vi "UHR-Fleezers Control (host) - 10.5.vi"() -> ()   [LabVIEW 2011] (continued)
      n139 = xnode "Read/Write Control"("FPGA VI Reference In"=w286, "error in"=w285, "+ phase"=w284, "+ phase (GI)"=w284, "+ phase (MCL)"=w284, "+ phase (APD Acq)"=w284, "+ phase (APD 1 Gate)"=w284, "+ phase (APD 2 Gate)"=w284, "+ phase (Green FB)"=w284, "+ phase (GI) 2"=w284) -> ("FPGA VI Reference Out"=w287:T19, "error out"=w288:errorcluster)
    }
    frame #3 {
      n140 = Wait (ms)(milliseconds to wait=u32 100) -> ()  [unwired: 1 out]
    }
  }
  n141 = local read "Phase adj. (Green FB)"() -> (w117:i16)
  n142 = local read "Phase adj. (GI) 2"() -> (w92:i16)
  n143 = local read "Phase adjust (MCL)"() -> (w174:i16)
  n144 = local read "Phase adj. (AI1)"() -> (w176:i16)
  n145 = local read "Phase adj. (GI)"() -> (w175:i16)
  n146 = xnode "Read/Write Control"("FPGA VI Reference In"=w142, "error in"=w143, "Phase count adjustment"=w176, "Phase count adjustment (GI)"=w175, "Phase count adjustment (MCL)"=w174, "Phase Count Adjustment (APD Acq)"="Phase Adj. (APD Acq)", "Phase count adjustment (APD 1 Gate)"="Phase Adj. (APD 1 Gate)", "Phase count adjustment (APD 2 Gate)"="Phase Adj. (APD 2 Gate)", "Phase count adjustment (Green FB)"=w117, "Phase count adjustment (GI) 2"=w92) -> ("FPGA VI Reference Out"=w78:T19, "error out"=w151:errorcluster)
  n147 = call "Initialize RF boards - interlace 3.vi"("error in"=w151, "FPGA VI Reference In"=w78) -> ("error out"=w149:errorcluster, "FPGA VI Reference Out"=w150:T19)
  n148 = call "set RF board frequency - interlace.vi"("Board 2 Frequency Limits"=w122, "Board 1 Frequency Limits"=w124, "error in"=w149, "FPGA VI Reference In"=w150, "Board 2 Frequency 3 (MHz)"="BD 2 Frequency 3 (MHz)", "Board 1 Frequency 3 (MHz)"="BD 1 Frequency 3 (MHz)", "Board 2 Frequency 2 (MHz)"="BD 2 Frequency 2 (MHz)", "Board 2 Frequency 1 (MHz)"="BD 2 Frequency 1 (MHz)", "Board 1 Frequency 2 (MHz)"="BD 1 Frequency 2 (MHz)", "Board 1 Frequency 1  (MHz)"="BD 1 Frequency 1 (MHz)") -> ("error out"=w252:errorcluster, "FPGA VI Reference Out"=w253:T19)
  n149 = call "set RF board amplitude - interlace.vi"("Board 2 Amplitude Limits"=w121, "Board 1 Amplitude Limits"=w123, "error in"=w252, "FPGA VI Reference In"=w253, "Board 2 Amplitude 3 (%)"="BD 2 Amplitude 3 (%)", "Board 1 Amplitude 3 (%)"="BD 1 Amplitude 3 (%)", "Board 2 Amplitude 2 (%)"="BD 2 Amplitude 2 (%)", "Board 2 Amplitude 1 (%)"="BD 2 Amplitude 1 (%)", "Board 1 Amplitude 2 (%)"="BD 1 Amplitude 2 (%)", "Board 1 Amplitude 1 (%)"="BD 1 Amplitude 1 (%)") -> ("error out"=w240:errorcluster, "FPGA VI Reference Out"=w241:T19)
  n150 = flat-sequence {
    tunnel: w241 -> [w300]
    tunnel: w240 -> [w299]
    tunnel: [w298] -> w245
    tunnel: [w297] -> w244
    tunnel: [w304] -> w243
    tunnel: w245 -> [w304]
    tunnel: [w303] -> w242
    tunnel: w244 -> [w303]
    tunnel: w243 -> [w313]
    tunnel: w242 -> [w312]
    tunnel: [w311] -> w40
    tunnel: [w310] -> w39
    frame #0 {
      n151 = local read "Trap 1 (ON/OFF)"() -> (w292:bool)
      n152 = xnode "Read/Write Control"("FPGA VI Reference In"=w300, "error in"=w299, "Direct RF Box  Communication"=FALSE) -> ("FPGA VI Reference Out"=w298:T19, "error out"=w297:errorcluster)
      n153 = local write "Saving..."(FALSE ("Saving Data")) -> ()
      n154 = local write "Stop All"(FALSE ("Stop All")) -> ()
      n155 = local write "Index"(1.0 ("Index")) -> ()
      n156 = property on="Trap 1 ON" class="Bool (strict)"("Value"=w292) -> ()  [unwired: 2 in, 2 out]
      "Manipulating Trap" <- FALSE ("Manipulating Trap")
    }
    frame #1 {
      n157 = local read "Trap 2 (ON/OFF)"() -> (w302:bool)
      n158 = Wait (ms)(milliseconds to wait=u32 10) -> ()  [unwired: 1 out]
      n159 = property on="Trap 2 ON" class="Bool (strict)"("Val(Sgnl)"=w302) -> ()  [unwired: 2 in, 2 out]
    }
    frame #2 {
      n160 = local read "Scan Range (nm)"() -> (w306:dbl)
      n161 = xnode "Read/Write Control"("FPGA VI Reference In"=w313, "error in"=w312, "FPGA Controls  RF Box"=TRUE ("Direct RF Box  Communication")) -> ("FPGA VI Reference Out"=w311:T19, "error out"=w310:errorcluster)
      n162 = call "Update messages.vi"("Message to add"="UHR-Fleezers ready.", "Old message string"="") -> ("New message string"=w309:string)
      n163 = local write "Messages"(w309) -> ()
      n164 = property on="Scan Range (nm)" class="DigNum (strict)"("Val(Sgnl)"=w306) -> ()  [unwired: 2 in, 2 out]
    }
  }
  n165 = Subtract(x="BD 1 Frequency 1 (MHz)", y="BD 1 Frequency 2 (MHz)") -> (x-y=w161:dbl)
  n166 = Subtract(x="BD 2 Frequency 1 (MHz)", y="BD 2 Frequency 2 (MHz)") -> (x-y=w160:dbl)
  n167 = Square(x=w160) -> (x^2=w158:dbl)
  n168 = Square(x=w161) -> (x^2=w159:dbl)
  n169 = Add(x=w159, y=w158) -> (x+y=w157:dbl)
  n170 = Square Root(x=w157) -> (sqrt(x)=w156:dbl)
  n171 = local write "Trap Delta (MHz)"(w156) -> ()
  n172 = call "IMAQ Create"("Image Name"="APD 1 Image", "Image Type"=w64) -> ("New Image"=w63:T3)  [unwired: 3 in, 1 out]
  n173 = call "IMAQ Create"("Image Name"="APD 2 Image", "Image Type"=w64) -> ("New Image"=w62:T3)  [unwired: 3 in, 1 out]
  n174 = call "IMAQ Create"("Image Name"="Det. X Image", "Image Type"=w64) -> ("New Image"=w61:T3)  [unwired: 3 in, 1 out]
  n175 = call "IMAQ Create"("Image Name"="Det. Y Image", "Image Type"=w64) -> ("New Image"=w60:T3)  [unwired: 3 in, 1 out]
  n176 = Bundle("New Image"=w63, "New Image"=w62, "New Image"=w61, "New Image"=w60) -> (w59:T20)  [unwired: 1 in]
  n177 = call-poly "VISA Configure Serial Port"("VISA resource name"="Sample Chamber Stage Serial Port") -> ("VISA resource name out"=w73:refnum<visa-resource-name>, "error out"=w74:errorcluster)  [unwired: 5 in, 8 out]
  "Stage Control Serial Error" <- w74
  n178 = call-poly "VISA Configure Serial Port"("VISA resource name"="Harvard Syringe Pump Serial Port", "baud rate (9600)"=u32 115200, "stop bits (10: 1 bit)"=w57) -> ("VISA resource name out"=w54:refnum<visa-resource-name>, "error out"=w55:errorcluster)  [unwired: 4 in, 7 out]
  n179 = node-c288() -> (w69:T21)  [unwired: 4 in]
  n180 = timed-loop "Run Scripts, including: stage motion" {
    tunnel: w74 -> [w317]
    tunnel: w73 -> [w318]
    tunnel: [w318] -> w72
    tunnel: [w317] -> w71
    timing: w69 -> [_]
    timing-out: [_] -> w68
    tunnel: w54 -> [w316]
    tunnel: w55 -> [w315]
    stop <- w319 stop-if-true
    n181 = node-c288() -> ()  [unwired: 1 in, 1 out]
    n182 = event shown="[3] \"Move Cap. 2 (ADig Top)\": Value Change" {
      selector: _ -> [_ _ _ _ _ _ _ _ _ _ _ _ _ _ _ _ _ _ _]
      dyn-events: _ -> [_ _ _ _ _ _ _ _ _ _ _ _ _ _ _ _ _ _ _]
      timeout: _ -> [_ _ _ _ _ _ _ _ _ _ _ _ _ _ _ _ _ _ _]
      tunnel: ["Set Position" "Move to Position" "Move Cap. 1 (DNA Bottom)" "Move Cap. 2 (ADig Top)" "Read Harvard" _ "Cal/Data Acq. Spot" "Dump Beads" _ _ _ "Got ADig bead" "Force FB Data\nScript" _ "Got DNA bead" "Take Stepping Data" _ "Take Detection Laser\nImage" _] -> _
      tunnel: [_ _ _ _ _ _ _ _ _ _ _ _ _ _ _ _ _ _ w946] -> w319
      tunnel: w317 -> [w337 w345 w359 w397 _ w443 w483 w571 w600 w728 w754 _ w791 _ _ _ _ _ _]
      tunnel: w318 -> [w338 w346 w360 w398 _ w444 w484 w572 w601 w729 w755 _ w792 _ _ _ _ _ _]
      tunnel: w316 -> [_ _ _ _ w428 _ _ _ _ _ _ _ _ _ _ _ _ _ _]
      tunnel: w315 -> [_ _ _ _ w427 _ _ _ _ _ _ _ _ _ _ _ _ _ _]
      event "Set Position", "Set Position 2", "Set Position 3", "Set Position 4", "Set Position 5", "Set Position 1": Value Change {
        n183 = event-data() -> ()  [unwired: 1 in, 5 out]
        n184 = Build Array("Set Position 1", "Set Position 2", "Set Position 3", "Set Position 4", "Set Position 5") -> (w336:bool[])
        n185 = Boolean Array To Number(Boolean array=w336) -> (number=w335:u32)
        n186 = Logarithm Base 2(1:w335) -> (0:w327:dbl)
        n187 = call "Read Stage Position.vi"("error in"=w337, "VISA resource name in"=w338) -> ("Current Position"=w342:cluster{dbl, dbl, dbl}, "error out"=w341:errorcluster)  [unwired: 2 out]
        n188 = Decrement(x="Position") -> (x-1=w325:dbl)
        n189 = Greater Or Equal?(x=w327, y=0.0) -> (x >= y?=w328:bool)
        n190 = Cluster To Array(cluster=w342) -> (array=w339:dbl[])
        n191 = local write "Stage Control Serial Error"(w341) -> ()
        n192 = Select(t=w327, s=w328, f=w325) -> (s? t:f=w324:dbl)
        n193 = Increment(x=w324) -> (x+1=w323:dbl)
        n194 = Build Array (concatenate)(w323, w339) -> (w322:dbl[])
        n195 = Replace Array Subset(array="Saved Stage Positions", new element=w322, index (row)=w324) -> (w340:dbl[][])  [unwired: 1 in]
        n196 = local write "Saved Stage Positions"(w340) -> ()
      }
      event "Move to Position": Value Change {
        n197 = event-data() -> ()  [unwired: 1 in, 5 out]
        n198 = flat-sequence {
          tunnel: w346 -> [w350]
          tunnel: w345 -> [w349]
          frame #0 {
            n199 = local read "Saved Stage Positions"() -> (w352:dbl[][])
            n200 = local read "Position"() -> (w351:dbl)
            n201 = local write "Stage Moving"(TRUE ("Stage Moving")) -> ()
            n202 = call "move to saved stage position.vi"("error in"=w349, "Stage VISA resource name in"=w350, "Position"=w351, "Saved Stage Positions"=w352) -> ("error out"=w348:errorcluster)  [unwired: 1 out]
            n203 = local write "Stage Control Serial Error"(w348) -> ()
          }
          frame #1 {
            n204 = call <vilib>:"Beep.vi"() -> ()  [unwired: 3 in, 9 out]
            n205 = local write "Stage Moving"(FALSE ("Stage Moving")) -> ()
          }
        }
      }
      event "Move Cap. 1 (DNA Bottom)": Value Change {
        n206 = event-data() -> ()  [unwired: 1 in, 5 out]
        n207 = local write "Move Cap. 1 (DNA Bottom)"(FALSE ("Move Cap. 1 (DNA Right)")) -> ()
        n208 = flat-sequence {
          tunnel: w359 -> [w366]
          tunnel: w360 -> [w367]
          tunnel: [w367] -> w357
          tunnel: [w366] -> w356
          tunnel: "Cap 1 Samp Flow ON" -> [w364]
          tunnel: w357 -> [w370]
          tunnel: w356 -> [w369]
          tunnel: "Cap 1 Samp Flow ON" -> [w383]
          frame #0 {
            n209 = local read "Sample Channel\nFlow"() -> (w365:bool)
            n210 = Not(x=w365) -> (.not. x?=w363:bool)
            n211 = And(x=w364, y=w363) -> (x .and. y?=w362:bool)
            n212 = case shown="True" w362 {
              frame False {
              }
              frame True {
                n213 = property on="Sample Channel\nFlow" class="Bool (strict)"("Val(Sgnl)"=TRUE ("Value (Signaling)")) -> ()  [unwired: 2 in, 2 out]
              }
            }
          }
          frame #1 {
            n214 = local read "Saved Stage Positions"() -> (w380:dbl[][])
            n215 = Array Subset(array=w380, index (row)=0 ("index"), length (row)=1 ("length"), index (col)=1 ("index"), length (col)=3 ("length")) -> (w377:dbl[][])
            n216 = local write "Stage Moving"(TRUE ("Stage Moving")) -> ()
            n217 = Reshape Array(w377, 3 ("dimension size")) -> (w375:dbl[])
            n218 = Array To Cluster(array=w375) -> (cluster=w374:cluster{"[0]":dbl, "[1]":dbl, "[2]":dbl})
            n219 = call "Set Stage Position.vi"("Position"=w374, "error in"=w369, "VISA resource name in"=w370) -> ("error out"=w373:errorcluster)  [unwired: 2 out]
            n220 = local write "Stage Control Serial Error"(w373) -> ()
          }
          frame #2 {
            n221 = local read "Sample Channel\nFlow"() -> (w384:bool)
            n222 = local write "Stage Moving"(FALSE ("Stage Moving")) -> ()
            n223 = call <vilib>:"Beep.vi"() -> ()  [unwired: 3 in, 9 out]
            n224 = And(x=w383, y=w384) -> (x .and. y?=w382:bool)
            n225 = case shown="True" w382 {
              frame False {
              }
              frame True {
                n226 = property on="Sample Channel\nFlow" class="Bool (strict)"("Val(Sgnl)"=FALSE ("Value (Signaling)")) -> ()  [unwired: 2 in, 2 out]
              }
            }
          }
          frame #3 {
            n227 = local read "Cap. 2 BD T1?\n(ADig T1, DNA T2)"() -> (w387:bool)
            n228 = case shown="True" "Cap 1 Flow ON" {
              frame False {
              }
              frame True {
                n229 = property on="Inject Pump 1" class="Bool (strict)"("Val(Sgnl)"=TRUE ("Value (Signaling)")) -> ()  [unwired: 2 in, 2 out]
              }
            }
            n230 = case shown="True" w387 {
              tunnel: "Cap 1 T ON" -> [w391 w392]
              frame False {
                n231 = property on="Trap 1 (ON/OFF)" class="Bool (strict)"("Val(Sgnl)"=w391) -> ()  [unwired: 2 in, 2 out]
              }
              frame True {
                n232 = property on="Trap 2 (ON/OFF)" class="Bool (strict)"("Val(Sgnl)"=w392) -> ()  [unwired: 2 in, 2 out]
              }
            }
          }
        }
      }
      event "Move Cap. 2 (ADig Top)": Value Change {
        n233 = event-data() -> ()  [unwired: 1 in, 5 out]
        n234 = local write "Move Cap. 2 (ADig Top)"(FALSE ("Move Cap. 2 (ADig Left)")) -> ()
        n235 = flat-sequence {
          tunnel: w397 -> [w401]
          tunnel: w398 -> [w402]
          tunnel: [w402] -> w395
          tunnel: [w401] -> w394
          tunnel: "Cap 2 Samp Flow ON" -> [w400]
          tunnel: w395 -> [w405]
          tunnel: w394 -> [w404]
          tunnel: "Cap 2 Samp Flow ON" -> [w417]
          frame #0 {
            n236 = case shown="True" w400 {
              frame False {
              }
              frame True {
                n237 = property on="Sample Channel\nFlow" class="Bool (strict)"("Val(Sgnl)"=TRUE ("Value (Signaling)")) -> ()  [unwired: 2 in, 2 out]
              }
            }
          }
          frame #1 {
            n238 = local read "Saved Stage Positions"() -> (w415:dbl[][])
            n239 = local write "Stage Moving"(TRUE ("Stage Moving")) -> ()
            n240 = Array Subset(array=w415, index (row)=1 ("index"), length (row)=1 ("length"), index (col)=1 ("index"), length (col)=3 ("length")) -> (w412:dbl[][])
            n241 = Reshape Array(w412, 3 ("dimension size")) -> (w410:dbl[])
            n242 = Array To Cluster(array=w410) -> (cluster=w409:cluster{"[0]":dbl, "[1]":dbl, "[2]":dbl})
            n243 = call "Set Stage Position.vi"("Position"=w409, "error in"=w404, "VISA resource name in"=w405) -> ("error out"=w408:errorcluster)  [unwired: 2 out]
            n244 = local write "Stage Control Serial Error"(w408) -> ()
          }
          frame #2 {
            n245 = case shown="True" w417 {
              frame False {
              }
              frame True {
                n246 = property on="Sample Channel\nFlow" class="Bool (strict)"("Val(Sgnl)"=FALSE ("Value (Signaling)")) -> ()  [unwired: 2 in, 2 out]
              }
            }
            n247 = local write "Stage Moving"(FALSE ("Stage Moving")) -> ()
            n248 = call <vilib>:"Beep.vi"() -> ()  [unwired: 3 in, 9 out]
          }
          frame #3 {
            n249 = case shown="True" "Cap 2 Flow ON" {
              frame False {
              }
              frame True {
                n250 = property on="Inject Pump 3" class="Bool (strict)"("Val(Sgnl)"=TRUE ("Value (Signaling)")) -> ()  [unwired: 2 in, 2 out]
              }
            }
            n251 = case shown="False" "Cap. 2 BD T1?\n(ADig T1, DNA T2)" {
              tunnel: "Cap 2 T ON" -> [w424 w425]
              frame False {
                n252 = property on="Trap 2 (ON/OFF)" class="Bool (strict)"("Val(Sgnl)"=w424) -> ()  [unwired: 2 in, 2 out]
              }
              frame True {
                n253 = property on="Trap 1 (ON/OFF)" class="Bool (strict)"("Val(Sgnl)"=w425) -> ()  [unwired: 2 in, 2 out]
              }
            }
          }
        }
      }
      event "Read Harvard": Value Change {
        n254 = event-data() -> ()  [unwired: 1 in, 5 out]
        n255 = Concatenate Strings("write buffer", "\r") -> (w430:string)
        n256 = VISA Write(VISA resource name=w428, write buffer=w430, error in (no error)=w427) -> (VISA resource name out=w439:refnum<visa-resource-name>, error out=w438:errorcluster)  [unwired: 1 out]
        n257 = stacked-sequence {
          tunnel: [w442] -> w437
          tunnel: w439 -> [w442]
          tunnel: w438 -> [w441]
          tunnel: [w441] -> w432
          frame #0 {
            n258 = Wait (ms)(milliseconds to wait=50) -> ()  [unwired: 1 out]
          }
        }
        n259 = property class="Instr"(reference=w437, error in=w432) -> (reference out=w436:refnum<visa-resource-name>, error out=w434:errorcluster, "Serial Settings:Number of Bytes at Serial Port"=w435:u32)
        "Serial Settings:Number of Bytes at Serial Port" <- w435
        n260 = VISA Read(VISA resource name=w436, byte count=w435, error in (no error)=w434) -> (read buffer=w433:string)  [unwired: 3 out]
        "read buffer" <- w433
        n261 = Fract/Exp String To Number(string=w433) -> ()  [unwired: 5 out]
      }
      event "+z", "-z": Value Change {
        n262 = event-data() -> ()  [unwired: 1 in, 5 out]
        n263 = flat-sequence {
          tunnel: w443 -> [w465]
          tunnel: w444 -> [w445]
          frame #0 {
            n264 = call "Read Stage Position.vi"("error in"=w465, "VISA resource name in"=w445) -> ("Current Position"=w450:cluster{dbl, dbl, dbl}, "error out"=w463:errorcluster, "VISA resource name out"=w464:refnum<visa-resource-name>)  [unwired: 1 out]
            n265 = local read "Saved Stage Positions"() -> (w474:dbl[][])
            n266 = Divide(x="z nudge increment (um)", y=1000.0) -> (x/y=w462:dbl)
            n267 = Boolean To (0,1)(Boolean="+z") -> (0, 1=w454:i16)
            n268 = Boolean To (0,1)(Boolean="-z") -> (0, 1=w455:i16)
            n269 = Array Subset(array=w474, index (row)=1 ("index"), length (row)=1 ("length"), index (col)=1 ("index"), length (col)=3 ("length")) -> (w471:dbl[][])
            n270 = Multiply(x=w454, y=w462) -> (x*y=w458:dbl)
            n271 = Multiply(x=w455, y=w462) -> (x*y=w456:dbl)
            n272 = Unbundle(w450) -> (w448:dbl, w447:dbl, w451:dbl)
            n273 = Negate(x=w456) -> (-x=w457:dbl)
            n274 = Reshape Array(w471, 3 ("dimension size")) -> (w469:dbl[])
            n275 = Add(x=w458, y=w457) -> (x+y=w459:dbl)
            n276 = Array To Cluster(array=w469) -> ()  [unwired: 1 out]
            n277 = Add(x=w459, y=w451) -> (x+y=w449:dbl)
            n278 = Bundle(cluster=w450, w448, w447, w449) -> (w446:cluster{dbl, dbl, dbl})
            n279 = call "Set Stage Position.vi"("Position"=w446, "error in"=w463, "VISA resource name in"=w464) -> ("error out"=w468:errorcluster)  [unwired: 2 out]
            n280 = local write "Stage Moving"(TRUE ("Stage Moving")) -> ()
            n281 = local write "Stage Control Serial Error"(w468) -> ()
          }
          frame #1 {
            n282 = local write "Stage Moving"(FALSE ("Stage Moving")) -> ()
            n283 = call <vilib>:"Beep.vi"() -> ()  [unwired: 3 in, 9 out]
          }
        }
      }
      event "Cal/Data Acq. Spot": Value Change {
        n284 = event-data() -> ()  [unwired: 1 in, 5 out]
        n285 = flat-sequence {
          tunnel: w483 -> [w491]
          tunnel: w484 -> [w492]
          tunnel: [w492] -> w480
          tunnel: [w491] -> w479
          tunnel: "Daq spot flow on" -> [w489]
          tunnel: w480 -> [w497]
          tunnel: w479 -> [w496]
          tunnel: ["Cal @ (MHz)"] -> w481
          tunnel: "Daq spot flow on" -> [w502]
          tunnel: w481 -> [w513]
          tunnel: ["W/ Offset 1"] -> w477
          tunnel: w481 -> [w534]
          tunnel: w477 -> [w532]
          frame #0 {
            n286 = local read "Sample Channel\nFlow"() -> (w488:bool)
            n287 = Not(x=w488) -> (.not. x?=w487:bool)
            n288 = And(x=w489, y=w487) -> (x .and. y?=w486:bool)
            n289 = case shown="True" w486 {
              frame False {
              }
              frame True {
                n290 = property on="Sample Channel\nFlow" class="Bool (strict)"("Val(Sgnl)"=TRUE ("Value (Signaling)")) -> ()  [unwired: 2 in, 2 out]
              }
            }
            n291 = Wait (ms)(milliseconds to wait=u32 250) -> ()  [unwired: 1 out]
          }
          frame #1 {
            n292 = local read "Saved Stage Positions"() -> (w494:dbl[][])
            n293 = local write "Stage Moving"(TRUE ("Stage Moving")) -> ()
            n294 = call "move to saved stage position.vi"("error in"=w496, "Stage VISA resource name in"=w497, "Position"="Cal Stage Position", "Saved Stage Positions"=w494) -> ("error out"=w495:errorcluster)  [unwired: 1 out]
            n295 = local write "Stage Control Serial Error"(w495) -> ()
          }
          frame #2 {
            n296 = property on="Trap Delta (MHz)" class="DigNum (strict)"("Val(Sgnl)"="Cal @ (MHz)") -> ()  [unwired: 2 in, 2 out]
            n297 = local read "Sample Channel\nFlow"() -> (w501:bool)
            n298 = local write "Stage Moving"(FALSE ("Stage Moving")) -> ()
            n299 = call <vilib>:"Beep.vi"() -> ()  [unwired: 3 in, 9 out]
            n300 = And(x=w502, y=w501) -> (x .and. y?=w500:bool)
            n301 = case shown="True" w500 {
              frame False {
              }
              frame True {
                n302 = property on="Sample Channel\nFlow" class="Bool (strict)"("Val(Sgnl)"=FALSE ("Value (Signaling)")) -> ()  [unwired: 2 in, 2 out]
              }
            }
          }
          frame #3 {
            n303 = Wait (ms)(milliseconds to wait=u32 500) -> ()  [unwired: 1 out]
          }
          frame #4 {
            n304 = property on="Save Calibration" class="Bool (strict)"("Val(Sgnl)"=TRUE ("Value (Signaling)")) -> ()  [unwired: 2 in, 2 out]
          }
          frame #5 {
            n305 = Wait (ms)(milliseconds to wait=u32 4000) -> ()  [unwired: 1 out]
          }
          frame #6 {
            n306 = while {
              stop <- w509 stop-if-true
              n307 = local read "Saving..."() -> (w510:bool)
              n308 = Wait (ms)(milliseconds to wait=u32 100) -> ()  [unwired: 1 out]
              n309 = Not(x=w510) -> (.not. x?=w509:bool)
            }
          }
          frame #7 {
            n310 = case shown="False" "W/ Offset 1" {
              tunnel: w513 -> [_ w514]
              frame False {
              }
              frame True {
                n311 = stacked-sequence {
                  tunnel: w514 -> [_ _ _ _ _ _ _ w531]
                  frame #0 {
                    n312 = property on="Trap Delta (MHz)" class="DigNum (strict)"("Val(Sgnl)"="Offset 1 Start (MHz)") -> ()  [unwired: 2 in, 2 out]
                    n313 = Replace Array Subset(array=u32[] [0] ("Index Values"), new element="Offset 1 Set", index=0) -> (w515:u32[])
                    n314 = property on="Saved AOD Raster Scan Parameter Sets" class="Arr (strict)"("Index Values"=w515) -> ()  [unwired: 2 in, 2 out]
                  }
                  frame #1 {
                    n315 = Wait (ms)(milliseconds to wait=u32 200) -> ()  [unwired: 1 out]
                  }
                  frame #2 {
                    n316 = property on="Load parameters" class="Bool (strict)"("Val(Sgnl)"=TRUE ("Value (Signaling)")) -> ()  [unwired: 2 in, 2 out]
                  }
                  frame #3 {
                    n317 = Wait (ms)(milliseconds to wait=u32 200) -> ()  [unwired: 1 out]
                  }
                  frame #4 {
                    n318 = property on="Trap Raster Scan" class="Bool (strict)"("Val(Sgnl)"=TRUE ("Value (Signaling)")) -> ()  [unwired: 2 in, 2 out]
                  }
                  frame #5 {
                    n319 = Wait (ms)(milliseconds to wait=u32 2000) -> ()  [unwired: 1 out]
                  }
                  frame #6 {
                    n320 = while {
                      stop <- w528 stop-if-true
                      n321 = local read "Raster Scanning..."() -> (w530:bool)
                      n322 = local read "Saving..."() -> (w526:bool)
                      n323 = Wait (ms)(milliseconds to wait=u32 100) -> ()  [unwired: 1 out]
                      n324 = Not(x=w526) -> (.not. x?=w525:bool)
                      n325 = Not(x=w530) -> (.not. x?=w527:bool)
                      n326 = And(x=w527, y=w525) -> (x .and. y?=w528:bool)
                    }
                  }
                  frame #7 {
                    n327 = property on="Trap Delta (MHz)" class="DigNum (strict)"("Val(Sgnl)"=w531) -> ()  [unwired: 2 in, 2 out]
                  }
                }
              }
            }
          }
          frame #8 {
            n328 = local read "Save ave N"() -> (w533:dbl)
            n329 = case shown="False" "W/ Offset 2" {
              tunnel: w534 -> [_ w541]
              tunnel: w533 -> [_ w540]
              tunnel: w532 -> [w536 _]
              frame False {
                n330 = case shown="False" w536 {
                  frame False {
                    n331 = Multiply(x="Cal read wait (s)", y=u32 1000 ("milliseconds to wait")) -> (x*y=w538:u32)
                    n332 = Wait (ms)(milliseconds to wait=w538) -> ()  [unwired: 1 out]
                  }
                  frame True {
                  }
                }
              }
              frame True {
                n333 = stacked-sequence {
                  tunnel: w541 -> [_ _ _ _ _ _ _ _ _ w562 _ _]
                  tunnel: w540 -> [_ _ _ _ _ _ _ _ _ w560 _ _]
                  frame #0 {
                    n334 = property on="Save ave N" class="DigNum (strict)"("Val(Sgnl)"=1.0 ("Value (Signaling)")) -> ()  [unwired: 2 in, 2 out]
                  }
                  frame #1 {
                    n335 = Wait (ms)(milliseconds to wait=u32 500) -> ()  [unwired: 1 out]
                  }
                  frame #2 {
                    n336 = property on="Trap Delta (MHz)" class="DigNum (strict)"("Val(Sgnl)"="Offset 2 Start (MHz)") -> ()  [unwired: 2 in, 2 out]
                    n337 = Replace Array Subset(array=u32[] [0] ("Index Values"), new element="Offset 2 Set", index=0) -> (w546:u32[])
                    n338 = property on="Saved AOD Raster Scan Parameter Sets" class="Arr (strict)"("Index Values"=w546) -> ()  [unwired: 2 in, 2 out]
                  }
                  frame #3 {
                    n339 = Wait (ms)(milliseconds to wait=u32 500) -> ()  [unwired: 1 out]
                  }
                  frame #4 {
                    n340 = property on="Load parameters" class="Bool (strict)"("Val(Sgnl)"=TRUE ("Value (Signaling)")) -> ()  [unwired: 2 in, 2 out]
                  }
                  frame #5 {
                    n341 = Wait (ms)(milliseconds to wait=u32 500) -> ()  [unwired: 1 out]
                  }
                  frame #6 {
                    n342 = property on="Trap Raster Scan" class="Bool (strict)"("Val(Sgnl)"=TRUE ("Value (Signaling)")) -> ()  [unwired: 2 in, 2 out]
                  }
                  frame #7 {
                    n343 = Wait (ms)(milliseconds to wait=u32 2000) -> ()  [unwired: 1 out]
                  }
                  frame #8 {
                    n344 = while {
                      stop <- w555 stop-if-true
                      n345 = local read "Raster Scanning..."() -> (w558:bool)
                      n346 = local read "Saving..."() -> (w556:bool)
                      n347 = Wait (ms)(milliseconds to wait=u32 100) -> ()  [unwired: 1 out]
                      n348 = Not(x=w556) -> (.not. x?=w554:bool)
                      n349 = Not(x=w558) -> (.not. x?=w557:bool)
                      n350 = And(x=w557, y=w554) -> (x .and. y?=w555:bool)
                    }
                  }
                  frame #9 {
                    n351 = property on="Trap Delta (MHz)" class="DigNum (strict)"("Val(Sgnl)"=w562) -> ()  [unwired: 2 in, 2 out]
                    n352 = property on="Saved AOD Raster Scan Parameter Sets" class="Arr (strict)"("Index Values"=u32[] [0]) -> ()  [unwired: 2 in, 2 out]
                    n353 = property on="Save ave N" class="DigNum (strict)"("Val(Sgnl)"=w560) -> ()  [unwired: 2 in, 2 out]
                  }
                  frame #10 {
                    n354 = Wait (ms)(milliseconds to wait=u32 500) -> ()  [unwired: 1 out]
                  }
                  frame #11 {
                    n355 = property on="Load parameters" class="Bool (strict)"("Val(Sgnl)"=TRUE ("Value (Signaling)")) -> ()  [unwired: 2 in, 2 out]
                  }
                }
              }
            }
          }
          frame #9 {
            n356 = property on="Read Cal" class="Bool (strict)"("Val(Sgnl)"=TRUE ("Value (Signaling)")) -> ()  [unwired: 2 in, 2 out]
          }
          frame #10 {
            n357 = Wait (ms)(milliseconds to wait=u32 1000) -> ()  [unwired: 1 out]
          }
          frame #11 {
            n358 = property on="Fish for Tether" class="Bool (strict)"("Val(Sgnl)"=TRUE ("Value (Signaling)")) -> ()  [unwired: 2 in, 2 out]
          }
        }
        n359 = local write "Cal/Data Acq. Spot"(FALSE ("Cal/Data Acq. Spot")) -> ()
      }
      event "Dump Beads": Value Change {
        n360 = event-data() -> ()  [unwired: 1 in, 5 out]
        n361 = flat-sequence {
          tunnel: ["Dump spot flow on?"] -> w568
          tunnel: [w579] -> w569
          tunnel: w568 -> [w579]
          tunnel: w572 -> [w584]
          tunnel: w571 -> [w583]
          tunnel: [w581] -> w570
          tunnel: w569 -> [w581]
          tunnel: w570 -> [w594]
          frame #0 {
            n362 = local read "Saving..."() -> (w575:bool)
            n363 = local write "Dump Beads"(FALSE ("Dump Beads")) -> ()
            n364 = local write "Stop Saving"(w575) -> ()
          }
          frame #1 {
            w576 = FALSE ("Fl. Triggered...")
            n365 = case shown="True" "Dump spot flow on?" {
              frame False {
              }
              frame True {
                n366 = property on="Sample Channel\nFlow" class="Bool (strict)"("Val(Sgnl)"=TRUE ("Stage Moving")) -> ()  [unwired: 2 in, 2 out]
              }
            }
            n367 = local write "Fl. Triggered..."(w576) -> ()
            n368 = local write "Tether"(w576) -> ()
            n369 = property on="Green Laser ON/Interlacing" class="Bool (strict)"("Val(Sgnl)"=w576) -> ()  [unwired: 2 in, 2 out]
            n370 = property on="Trap Pos. FB ON" class="Bool (strict)"("Val(Sgnl)"=w576) -> ()  [unwired: 2 in, 2 out]
            n371 = property on="Trap Trig. Fl." class="Bool (strict)"("Val(Sgnl)"=w576) -> ()  [unwired: 2 in, 2 out]
            n372 = property on="Dip for Protein" class="Bool (strict)"("Val(Sgnl)"=w576) -> ()  [unwired: 2 in, 2 out]
            n373 = property on="Pause dwell \ntimer" class="Bool (strict)"("Val(Sgnl)"=w576) -> ()  [unwired: 2 in, 2 out]
          }
          frame #2 {
            n374 = property on="Trap Pos. FB Offset Factor" class="DigNum (strict)"("Val(Sgnl)"=i64 0 ("Value (Signaling)")) -> ()  [unwired: 2 in, 2 out]
          }
          frame #3 {
            n375 = local read "Saved Stage Positions"() -> (w585:dbl[][])
            n376 = local write "Stage Moving"(TRUE ("Stage Moving")) -> ()
            n377 = Array Subset(array=w585, index (row)=3 ("index"), length (row)=1 ("length"), index (col)=1 ("index"), length (col)=3 ("length")) -> (w590:dbl[][])
            n378 = Reshape Array(w590, 3 ("dimension size")) -> (w588:dbl[])
            n379 = Array To Cluster(array=w588) -> (cluster=w587:cluster{"[0]":dbl, "[1]":dbl, "[2]":dbl})
            n380 = call "Set Stage Position.vi"("Position"=w587, "error in"=w583, "VISA resource name in"=w584) -> ()  [unwired: 3 out]
          }
          frame #4 {
            w595 = FALSE ("Value (Signaling)")
            n381 = case shown="True" w594 {
              frame False {
              }
              frame True {
                n382 = property on="Sample Channel\nFlow" class="Bool (strict)"("Val(Sgnl)"=FALSE ("Stage Moving")) -> ()  [unwired: 2 in, 2 out]
              }
            }
            n383 = property on="Trap 1 (ON/OFF)" class="Bool (strict)"("Val(Sgnl)"=w595) -> ()  [unwired: 2 in, 2 out]
            n384 = property on="Trap 2 (ON/OFF)" class="Bool (strict)"("Val(Sgnl)"=w595) -> ()  [unwired: 2 in, 2 out]
            n385 = call <vilib>:"Beep.vi"() -> ()  [unwired: 3 in, 9 out]
          }
          frame #5 {
            n386 = property on="Move Cap. 2 (ADig Top)" class="Bool (strict)"("Val(Sgnl)"=TRUE ("Value (Signaling)")) -> ()  [unwired: 2 in, 2 out]
            n387 = property on="Tab Control" class="TabCtl (strict)"("Val(Sgnl)"=T5."Status" ("Value (Signaling)")) -> ()  [unwired: 2 in, 2 out]
          }
        }
      }
      event "Dip for Protein": Value Change {
        n388 = event-data() -> ()  [unwired: 1 in, 5 out]
        n389 = case shown="True" "Dip for Protein" {
          tunnel: w601 -> [_ w603]
          tunnel: w600 -> [_ w602]
          frame False {
          }
          frame True {
            n390 = while {
              tunnel: w603 -> [w614]
              tunnel: w602 -> [w613]
              i -> [w608]
              stop <- w610 stop-if-true
              n391 = Increment(x=w608) -> (x+1=→"Dip #":i32)
              n392 = flat-sequence {
                tunnel: w613 -> [w625]
                tunnel: w614 -> [w626]
                tunnel: [w626] -> w618
                tunnel: [w625] -> w617
                tunnel: [w619] -> w604
                tunnel: [w631] -> w612
                tunnel: [w632] -> w611
                tunnel: w618 -> [w633]
                tunnel: w617 -> [w634]
                tunnel: [w629] -> w605
                tunnel: w604 -> [w629]
                tunnel: [w642] -> w616
                tunnel: w612 -> [w642]
                tunnel: [w641] -> w615
                tunnel: w611 -> [w641]
                tunnel: [w638] -> w609
                tunnel: [w637] -> w606
                tunnel: w605 -> [w637]
                tunnel: w615 -> [w663]
                tunnel: w616 -> [w664]
                tunnel: w609 -> [w665]
                tunnel: w606 -> [w662]
                tunnel: [w716] -> w610
                frame #0 {
                  n393 = local read "Trap Pos. FB ON"() -> (w619:bool)
                  n394 = Compound Arithmetic op=AND("Flow ON\nduring dip?", "FB OFF when \nflow ON", w619) -> (w620:bool)
                  n395 = case shown="True" "Move trap \nbefore dip move?" {
                    frame False {
                    }
                    frame True {
                      n396 = property on="Trap Delta (MHz)" class="DigNum (strict)"("Val(Sgnl)"="Dipping Delta (MHz)") -> ()  [unwired: 2 in, 2 out]
                    }
                  }
                  n397 = property on="Green Laser ON/Interlacing" class="Bool (strict)"("Val(Sgnl)"="Green ON\nbefore dip?") -> ()  [unwired: 2 in, 2 out]
                  n398 = property on="Sample Channel\nFlow" class="Bool (strict)"("Val(Sgnl)"="Flow ON\nduring dip?") -> ()  [unwired: 2 in, 2 out]
                  n399 = case shown="True" w620 {
                    frame False {
                    }
                    frame True {
                      n400 = property on="Trap Pos. FB ON" class="Bool (strict)"("Val(Sgnl)"=FALSE ("Value (Signaling)")) -> ()  [unwired: 2 in, 2 out]
                    }
                  }
                }
                frame #1 {
                  n401 = local read "Saved Stage Positions"() -> (w636:dbl[][])
                  n402 = local write "Cancel dwell"(FALSE ("Cancel dwell")) -> ()
                  n403 = call "move to saved stage position.vi"("error in"=w634, "Stage VISA resource name in"=w633, "Position"="Dip Stage \nPosition", "Saved Stage Positions"=w636) -> ("VISA resource name out"=w631:refnum<visa-resource-name>, "error out"=w632:errorcluster)
                }
                frame #2 {
                  n404 = node-c288() -> (w640:T21)  [unwired: 4 in]
                  n405 = timed-loop {
                    timing: w640 -> [_]
                    timing-out: [_] -> w639
                    tunnel: [w646] -> w638
                    i -> [w657]
                    stop <- w647 stop-if-true
                    n406 = node-c288() -> ()  [unwired: 1 in, 1 out]
                    n407 = Increment(x=w657) -> (x+1=→"Dip Time (s)":i32)
                    n408 = Greater Or Equal?(x=w657, y="Dip Duration (s)") -> (x >= y?=w655:bool)
                    n409 = local read "Dip for Protein"() -> (w648:bool)
                    n410 = local read "Dump Beads"() -> (w645:bool)
                    n411 = local read "Cancel dwell"() -> (w654:bool)
                    n412 = local read "Pause dwell \ntimer"() -> (w651:bool)
                    n413 = Not(x=w648) -> (.not. x?=w653:bool)
                    n414 = Compound Arithmetic op=OR(w654, w655, w653) -> (w652:bool)
                    n415 = Select(t=FALSE, s=w651, f=w652) -> (s? t:f=w649:bool)
                    n416 = Not(x=w645) -> (.not. x?=w644:bool)
                    n417 = node-c288() -> ()  [unwired: 1 in, 1 out]
                    n418 = And(x=w648, y=w644) -> (x .and. y?=w646:bool)
                    n419 = Or(x=w649, y=w645) -> (x .or. y?=w647:bool)
                  }
                  n420 = node-c288(w639) -> ()  [unwired: 1 out]
                }
                frame #3 {
                  n421 = case shown="True" w665 {
                    tunnel: w664 -> [_ w670]
                    tunnel: w663 -> [_ w669]
                    tunnel: w662 -> [_ w666]
                    frame False {
                    }
                    frame True {
                      n422 = flat-sequence {
                        tunnel: w669 -> [w674]
                        tunnel: w670 -> [w675]
                        tunnel: [w675] -> w668
                        tunnel: [w674] -> w667
                        tunnel: w666 -> [w671]
                        tunnel: w668 -> [w684]
                        tunnel: w667 -> [w683]
                        tunnel: w666 -> [w688]
                        frame #0 {
                          n423 = local read "Sample Channel\nFlow"() -> (w673:bool)
                          n424 = case shown="True" w673 {
                            tunnel: "Flow ON \nduring return\nfrom dip?" -> [w676 w679]
                            tunnel: w671 -> [_ w678]
                            frame False {
                              n425 = case shown="False" w676 {
                                frame False {
                                }
                                frame True {
                                n426 = property on="Sample Channel\nFlow" class="Bool (strict)"("Val(Sgnl)"=TRUE ("Value (Signaling)")) -> ()  [unwired: 2 in, 2 out]
                                }
                              }
                            }
                            frame True {
                              n427 = case shown="False" w679 {
                                tunnel: w678 -> [w680 _]
                                frame False {
                                n428 = property on="Trap Pos. FB ON" class="Bool (strict)"("Val(Sgnl)"=w680) -> ()  [unwired: 2 in, 2 out]
                                n429 = property on="Sample Channel\nFlow" class="Bool (strict)"("Val(Sgnl)"=FALSE ("Value (Signaling)")) -> ()  [unwired: 2 in, 2 out]
                                }
                                frame True {
                                }
                              }
                            }
                          }
                        }
                        frame #1 {
                          n430 = local read "Saved Stage Positions"() -> (w687:dbl[][])
                          n431 = local write "Cancel dwell"(FALSE ("Cancel dwell")) -> ()
                          n432 = call "move to saved stage position.vi"("error in"=w683, "Stage VISA resource name in"=w684, "Position"="Return Stage \nPosition", "Saved Stage Positions"=w687) -> ("error out"=w685:errorcluster)  [unwired: 1 out]
                          n433 = local write "Stage Control Serial Error"(w685) -> ()
                        }
                        frame #2 {
                          n434 = property on="Trap Pos. FB ON" class="Bool (strict)"("Val(Sgnl)"=w688) -> ()  [unwired: 2 in, 2 out]
                          n435 = case shown="True" "Green ON \nafter return?" {
                            frame False {
                            }
                            frame True {
                              n436 = property on="Green Laser ON/Interlacing" class="Bool (strict)"("Val(Sgnl)"=TRUE ("Value (Signaling)")) -> ()  [unwired: 2 in, 2 out]
                            }
                          }
                          n437 = case shown="True" "Move trap \nafter return move?" {
                            frame False {
                            }
                            frame True {
                              n438 = property on="Trap Delta (MHz)" class="DigNum (strict)"("Val(Sgnl)"="Dip Trap Delta 2 (MHz)") -> ()  [unwired: 2 in, 2 out]
                            }
                          }
                          n439 = case shown="True" "Save data\nafter return move?" {
                            frame False {
                            }
                            frame True {
                              n440 = property on="Start Saving" class="Bool (strict)"("Val(Sgnl)"=TRUE ("Value (Signaling)")) -> ()  [unwired: 2 in, 2 out]
                            }
                          }
                          n441 = property on="Sample Channel\nFlow" class="Bool (strict)"("Val(Sgnl)"="Flow ON\nduring daq?") -> ()  [unwired: 2 in, 2 out]
                        }
                        frame #3 {
                          n442 = node-c288() -> (w697:T21)  [unwired: 4 in]
                          n443 = timed-loop {
                            timing: w697 -> [_]
                            timing-out: [_] -> w696
                            i -> [w709]
                            stop <- w699 stop-if-true
                            n444 = node-c288() -> ()  [unwired: 1 in, 1 out]
                            n445 = local read "Dump Beads"() -> (w698:bool)
                            n446 = Greater Or Equal?(x=w709, y="Dwell Duration (s)") -> (x >= y?=w704:bool)
                            n447 = local read "Dip for Protein"() -> (w701:bool)
                            n448 = Not(x=w701) -> (.not. x?=w700:bool)
                            n449 = Compound Arithmetic op=OR(w704, "Cancel dwell", w700) -> (w703:bool)
                            n450 = node-c288() -> ()  [unwired: 1 in, 1 out]
                            n451 = Select(t=FALSE, s="Pause dwell \ntimer", f=w703) -> (s? t:f=w706:bool)
                            n452 = Or(x=w706, y=w698) -> (x .or. y?=w699:bool)
                          }
                          n453 = node-c288(w696) -> ()  [unwired: 1 out]
                        }
                      }
                    }
                  }
                }
                frame #4 {
                  n454 = local read "Dip for Protein"() -> (w717:bool)
                  n455 = local read "Dump Beads"() -> (w714:bool)
                  n456 = local write "Cancel dwell"(FALSE ("Cancel dwell")) -> ()
                  n457 = Not(x=w717) -> (.not. x?=w718:bool)
                  n458 = Not(x="Cont. Repeat Dipping?") -> (.not. x?=w720:bool)
                  n459 = Compound Arithmetic op=OR(w718, w720, w714) -> (w716:bool)
                }
              }
            }
          }
        }
      }
      event "Profile": Value Change {
        n460 = event-data() -> ()  [unwired: 1 in, 5 out]
        n461 = flat-sequence {
          tunnel: w729 -> [w732]
          tunnel: w728 -> [w740]
          tunnel: [w734] -> w727
          tunnel: [w733] -> w726
          tunnel: [w731] -> w724
          tunnel: [w730] -> w721
          tunnel: w727 -> [w747]
          tunnel: w726 -> [w746]
          tunnel: [w744] -> w725
          tunnel: w724 -> [w745]
          tunnel: [w743] -> w723
          tunnel: [w742] -> w722
          tunnel: w721 -> [w742]
          tunnel: w725 -> [w751]
          tunnel: w723 -> [w750]
          tunnel: w722 -> [w749]
          frame #0 {
            n462 = call "Read Stage Position.vi"("error in"=w740, "VISA resource name in"=w732) -> ("Current Position"=w730:cluster{dbl, dbl, dbl}, "error out"=w733:errorcluster, "VISA resource name out"=w731:refnum<visa-resource-name>)  [unwired: 1 out]
            "Current Position" <- w730
            n463 = local write "Stage Control Serial Error"(w733) -> ()
            n464 = Unbundle(w730) -> (w737:dbl, w739:dbl, w735:dbl)
            n465 = Add(x=w739, y="Y change (mm)") -> (x+y=w736:dbl)
            n466 = Bundle(w737, w736, w735) -> (w734:cluster{dbl, dbl, dbl})  [unwired: 1 in]
          }
          frame #1 {
            # "move to new position and start saving"
            n467 = local write "Stage Moving"(TRUE ("Stage Moving")) -> ()
            n468 = local write "Start Saving"(TRUE ("Start Saving")) -> ()
            n469 = call "Set Stage Position.vi"("Position"=w747, "error in"=w746, "VISA resource name in"=w745) -> ("error out"=w743:errorcluster, "VISA resource name out"=w744:refnum<visa-resource-name>)  [unwired: 1 out]
          }
          frame #2 {
            # "go back to start"
            n470 = call "Set Stage Position.vi"("Position"=w749, "error in"=w750, "VISA resource name in"=w751) -> ()  [unwired: 3 out]
          }
          frame #3 {
            # "stop saving"
            n471 = local write "Stop Saving"(TRUE ("Stop Saving")) -> ()
            n472 = local write "Stage Moving"(FALSE ("Stage Moving")) -> ()
          }
        }
      }
      event "Move to Position 1", "Move to Position 2", "Move to Position 3", "Move to Position 4", "Move to Position 5", "Lower Ch. Cap.": Value Change {
        n473 = event-data() -> ()  [unwired: 1 in, 5 out]
        n474 = Or(x="Move to Position 5", y="Lower Ch. Cap.") -> (x .or. y?=w757:bool)
        n475 = Build Array("Move to Position 1", "Move to Position 2", "Move to Position 3", "Move to Position 4", w757) -> (w760:bool[])
        n476 = Boolean Array To Number(Boolean array=w760) -> (number=w759:u32)
        n477 = Logarithm Base 2(1:w759) -> (0:w758:dbl)
        n478 = flat-sequence {
          tunnel: w758 -> [w769]
          tunnel: w755 -> [w767]
          tunnel: w754 -> [w766]
          frame #0 {
            n479 = local read "Saved Stage Positions"() -> (w777:dbl[][])
            n480 = Array Subset(array=w777, index (row)=w769, length (row)=1 ("length"), index (col)=1 ("index"), length (col)=3 ("length")) -> (w774:dbl[][])
            n481 = Reshape Array(w774, 3 ("dimension size")) -> (w772:dbl[])
            n482 = Array To Cluster(array=w772) -> (cluster=w771:cluster{"[0]":dbl, "[1]":dbl, "[2]":dbl})
            n483 = call "Set Stage Position.vi"("Position"=w771, "error in"=w766, "VISA resource name in"=w767) -> ("error out"=w770:errorcluster)  [unwired: 2 out]
            n484 = local write "Stage Moving"(TRUE ("Stage Moving")) -> ()
            n485 = local write "Stage Control Serial Error"(w770) -> ()
          }
          frame #1 {
            n486 = local write "Stage Moving"(FALSE ("Stage Moving")) -> ()
            n487 = call <vilib>:"Beep.vi"() -> ()  [unwired: 3 in, 9 out]
          }
        }
      }
      event "Got ADig bead": Value Change {
        n488 = event-data() -> ()  [unwired: 1 in, 5 out]
        n489 = local read "Cap 1 Samp Flow ON"() -> (w780:bool)
        n490 = flat-sequence {
          tunnel: w780 -> [w782]
          frame #0 {
            n491 = case shown="True" w782 {
              frame False {
              }
              frame True {
                n492 = property on="Sample Channel\nFlow" class="Bool (strict)"("Val(Sgnl)"=TRUE ("Value (Signaling)")) -> ()  [unwired: 2 in, 2 out]
              }
            }
          }
          frame #1 {
            n493 = property on="Move Cap. 1 (DNA Bottom)" class="Bool (strict)"("Val(Sgnl)"=TRUE ("Value (Signaling)")) -> ()  [unwired: 2 in, 2 out]
            n494 = property on="Inject Pump 3" class="Bool (strict)"("Val(Sgnl)"=FALSE ("Value (Signaling)")) -> ()  [unwired: 2 in, 2 out]
          }
        }
      }
      event "Force FB Data\nScript": Value Change {
        n495 = event-data() -> ()  [unwired: 1 in, 5 out]
        n496 = flat-sequence {
          tunnel: w791 -> [w795]
          tunnel: w792 -> [w796]
          tunnel: [w796] -> w787
          tunnel: [w795] -> w786
          tunnel: w787 -> [w799]
          tunnel: w786 -> [w798]
          tunnel: ["Trap Trig Fl."] -> w788
          tunnel: [w824] -> w789
          tunnel: w788 -> [w824]
          tunnel: [w827] -> w790
          tunnel: w789 -> [w827]
          tunnel: w790 -> [w830]
          frame #0 {
            n497 = property on="Trap Delta (MHz)" class="DigNum (strict)"("Val(Sgnl)"="Trap Delta Before Moving") -> ()  [unwired: 2 in, 2 out]
          }
          frame #1 {
            n498 = local read "Saved Stage Positions"() -> (w801:dbl[][])
            n499 = local write "FB Trap Pos Offset"(0.0 ("FB Trap Pos Offset")) -> ()
            n500 = property on="Trap Pos. FB Offset Factor" class="DigNum (strict)"("Val(Sgnl)"=i64 0 ("Value (Signaling)")) -> ()  [unwired: 2 in, 2 out]
            n501 = local write "Stage Moving"(TRUE ("Stage Moving")) -> ()
            n502 = call "move to saved stage position.vi"("error in"=w798, "Stage VISA resource name in"=w799, "Position"="Stage Position To Establish FB", "Saved Stage Positions"=w801) -> ("error out"=w797:errorcluster)  [unwired: 1 out]
            n503 = local write "Stage Control Serial Error"(w797) -> ()
          }
          frame #2 {
            n504 = call <vilib>:"Beep.vi"() -> ()  [unwired: 3 in, 9 out]
            n505 = Multiply(x="Wait (s)", y=u32 1000 ("milliseconds to wait")) -> (x*y=w807:u32)
            n506 = property on="Trap Delta (MHz)" class="DigNum (strict)"("Val(Sgnl)"="Starting \nTrap Delta (MHz)") -> ()  [unwired: 2 in, 2 out]
            n507 = local write "Stage Moving"(FALSE ("Stage Moving")) -> ()
            n508 = Wait (ms)(milliseconds to wait=w807) -> ()  [unwired: 1 out]
            n509 = property on="Tab Control 2" class="TabCtl (strict)"("Val(Sgnl)"=T6."Feedback on Trap Position" ("Value (Signaling)")) -> ()  [unwired: 2 in, 2 out]
            n510 = property on="Tab Control" class="TabCtl (strict)"("Val(Sgnl)"=T5."Trap Control (RF)" ("Value (Signaling)")) -> ()  [unwired: 2 in, 2 out]
          }
          frame #3 {
            n511 = property on="Set Reading to\nSetpoint" class="Bool (strict)"("Val(Sgnl)"=TRUE ("Value (Signaling)")) -> ()  [unwired: 2 in, 2 out]
            n512 = Wait (ms)(milliseconds to wait=u32 500) -> ()  [unwired: 1 out]
